vi "Get Account Info.vi"(8 "error in":errorcluster, 11 "PIN":string) -> (0 "error out":errorcluster, 1 "Verified?":bool, 2 "Account Balance":string, 3 "Account Name":string)   [LabVIEW 2025]
doc: "Retrieve the account information of the PIN provided if the PIN is verified."
uses:
  <vilib>/Utility/file.llb/Read Delimited Spreadsheet (string).vi
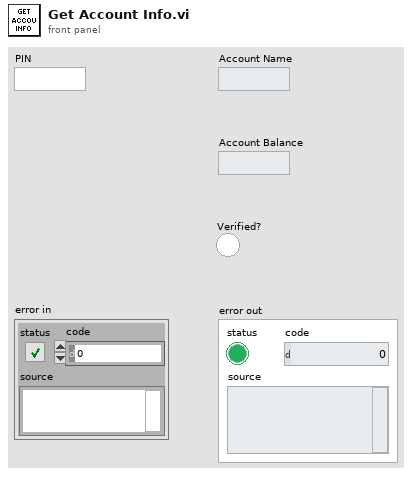
[diagram p1: front panel]
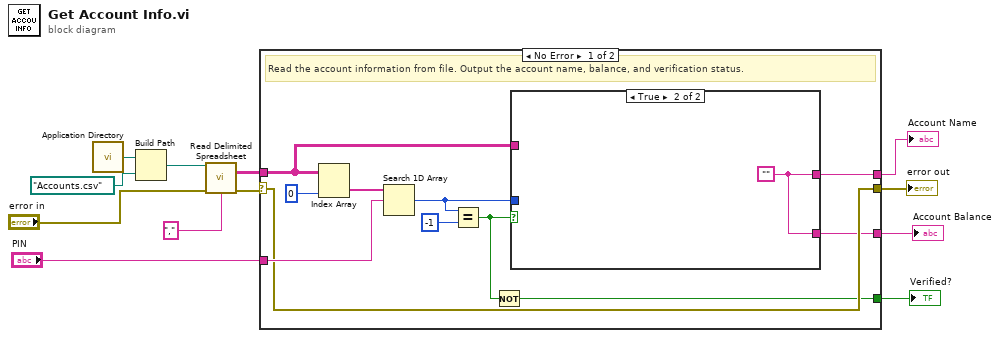
[diagram p0: block diagram]
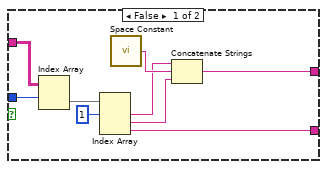
[diagram p2: hidden frame]
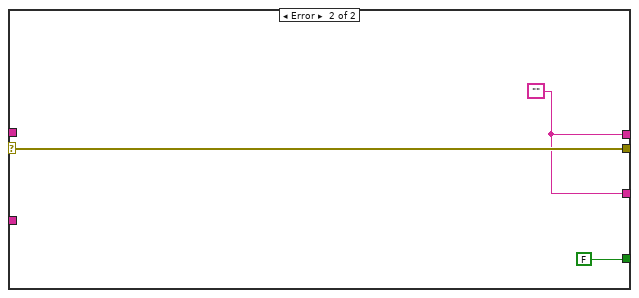
[diagram p3: hidden frame]
diagram:
  n1 = call <vilib>:"Application Directory.vi"() -> ("Application Directory"=w8:path)
  n2 = Build Path(base path=w8, name or relative path=path "Accounts.csv") -> (appended path=w10:path)
  n3 = call-poly <vilib>:"Read Delimited Spreadsheet.vi"("file path (dialog if empty)"=w10, "error in (no error)"="error in", "delimiter (\\t)"="," ("delimiter (\\t)")) -> ("all rows"=w12:string[][], "error out"=w5:errorcluster)  [unwired: 7 in, 4 out]
  n4 = case shown="No Error" w5 {
    selector: w5 -> [w17 w36]
    tunnel: w12 -> [w21 _]
    tunnel: "PIN" -> [w20 _]
    tunnel: [w17 w36] -> w4
    tunnel: [w15 FALSE] -> w3
    tunnel: [w14 w35] -> w2
    tunnel: [w13 w35] -> w1
    frame No Error {
      # "Read the account information from file. Output the account name, balance, and verification status."
      n5 = Index Array(array=w21, index (col)=0) -> (element=w19:string[])  [unwired: 1 in]
      n6 = Search 1D Array(1D array=w19, element=w20) -> (index of element=w22:i32)  [unwired: 1 in]
      n7 = Equal?(x=w22, y=-1) -> (x = y?=w16:bool)
      n8 = Not(x=w16) -> (.not. x?=w15:bool)
      n9 = case shown="True" w16 {
        tunnel: w21 -> [w32 _]
        tunnel: w22 -> [w31 _]
        tunnel: [w25 w33] -> w14
        tunnel: [w24 w33] -> w13
        frame False {
          n10 = Index Array(array=w32, index (row)=w31) -> (element=w30:string[])  [unwired: 1 in]
          n11 = Index Array(array=w30, index #1=1 ("index")) -> (element #1=w27:string, element #2=w26:string, element #3=w24:string)  [unwired: 2 in]
          n12 = call <vilib>:"Space Constant.vi"() -> ("String"=w28:string)
          n13 = Concatenate Strings(w27, w28, w26) -> (w25:string)
        }
        frame True {
          w33 = ""
        }
      }
    }
    frame Error {
      w35 = ""
    }
  }
  "error out" <- w4
  "Verified?" <- w3
  "Account Name" <- w2
  "Account Balance" <- w1
